vi "Init_Joint.vi"(7 "error in":errorcluster, 10 "X-CAN Session in":refnum<class "X-CAN.lvclass">) -> (0 "error out":errorcluster, 1 "Initial position":dbl[](array[numeric]), 2 "Init Position":T1(array[cluster]) {"Error Code" format="%b"; "ID" format="%x"}, 3 "X-CAN Session out":refnum<class "X-CAN.lvclass">)   [LabVIEW 2015]
uses:
  <vilib>/Stratom, Inc/X-CAN for myRIO (API)/X-CAN Class/X-CAN.lvclass
  <vilib>/Platform/TimedLoop/XDataNode/timing_clust.ctl
  <vilib>/Platform/TimedLoop/XDataNode/nitl_modes.ctl
  <vilib>/Platform/TimedLoop/XDataNode/wakeup.ctl
  <vilib>/Stratom, Inc/X-CAN for myRIO (API)/X-CAN Class/Type Definitions/CANFrame.ctl
  <vilib>/platform/TimedLoop/XDataNode/XDataNode.xnode
  <vilib>/Platform/TimedLoop/XDataNode/XDNodeRunTimeDep.lvlib
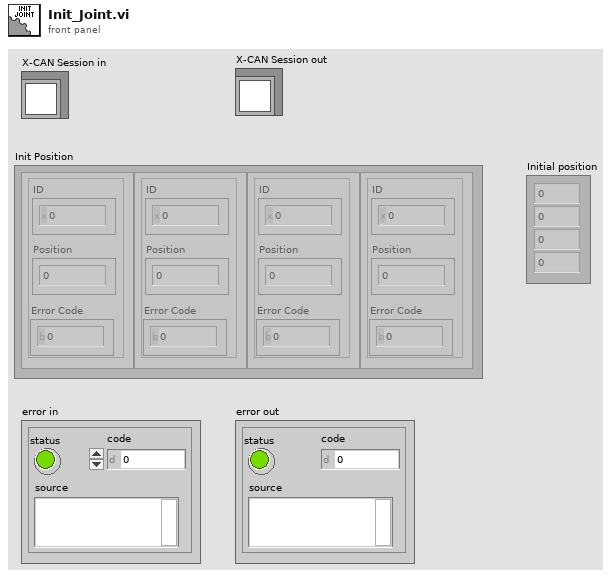
[diagram p1: front panel]
types:
  T1 = cluster{"ID":u8, "Position":u16, "Error Code":u8}[]
  T2 = typedef "XDNodeRunTimeDep.lvlib/timing_clust.ctl" = cluster{"Expected End [f-1]":u64, "Actual End [f-1]":u64, "Finished Late? [f-1]":bool, "Expected End [i-1]":u64, "Actual End [i-1]":u64, "Finished Late? [i-1]":bool, "Expected Start [i]":u64, "Actual Start [i]":u64, "Expected Start [f]":u64, "Actual Start [f]":u64, "Source Name":string, "Structure Name":string, "Period":i64, "Deadline":i64, "Offset":i64, "Start":i64, "Priority":i32, "Timeout":i32, "Mode":T3, "Wakeup Reason":T4, "Error":errorcluster, "Source Type":string, "Secondary Source Type":string, "Global End Time":u64, "Global Start Time":u64, "Frame Duration":u64, "Iteration Duration":u64, "Assigned CPU":i32, "I/O Scan Engine Mode":u32}
  T3 = typedef "XDNodeRunTimeDep.lvlib/nitl_modes.ctl" = enum32{"No Change", "Process missed periods, maintain original phase", "Discard missed periods, maintain original phase", "Process missed periods, ignore original phase", "Discard missed periods, ignore original phase"}
  T4 = typedef "XDNodeRunTimeDep.lvlib/wakeup.ctl" = enum32{"Normal", "Aborted", "Asynchronous wakeup", "Timing source error", "Timed loop error", "Timeout"}
  T5 = typedef "X-CAN.lvclass/CANFrame.ctl" = cluster{"identifier":u32, "extended?":bool, "echo?":bool, "payload":u8[], "timestamp":timestamp}
  T6 = cluster{"Error Code":u8, "Position":u16, "ID":u8}
  T7 = cluster{"ID":u8, "Position":u16, "Error Code":u8}
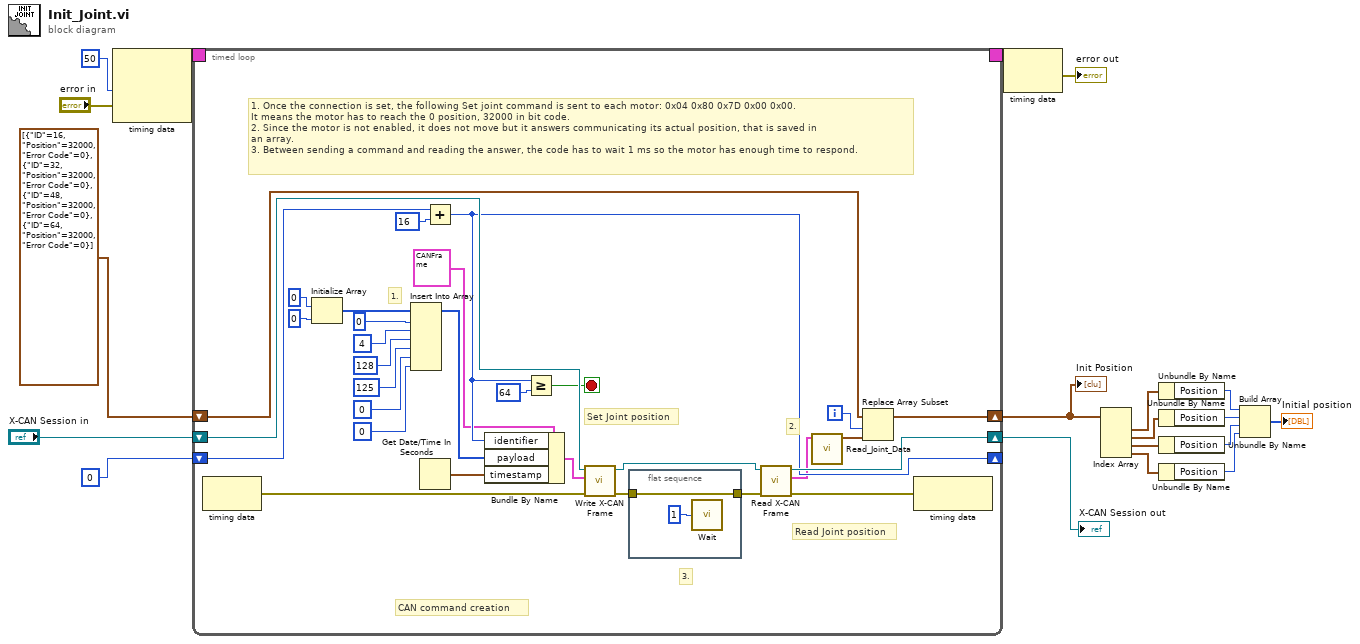
[diagram p0: block diagram]
diagram:
  n1 = node-c288(i64 50 ("Period"), "error in") -> (w19:T2)  [unwired: 1 in]
  n2 = timed-loop {
    timing: w19 -> [_]
    timing-out: [_] -> w18
    shift-right: [w49] -> w13
    shift-left: "X-CAN Session in" -> [w48]
    shift-right: [w47] -> _
    shift-left: u8 0 -> [w46]
    shift-right: [w45] -> w1
    shift-left: T1 [{"ID"=16, "Position"=32000, "Error Code"=0}, {"ID"=32, "Position"=32000, "Error Code"=0}, {"ID"=48, "Position"=32000, "Error Code"=0}, {"ID"=64, "Position"=32000, "Error Code"=0}] ("Array") -> [w44]
    i -> [w40]
    stop <- w41 stop-if-true
    # "1. Once the connection is set, the following Set joint command is sent to each motor: 0x04 0x80 0x7D 0x00 0x00.\nIt means the motor has to reach the 0 position, 32000 in bit code.\n2. Since the motor is not enabled, it does not move but it answers communicating its actual position, that is saved in\nan array.\n3. Between sending a command and reading the answer, the code has to wait 1 ms so the motor has enough time to respond."
    # "Read Joint position"
    # "3."
    # "2."
    # "1."
    # "Set Joint position"
    # "CAN command creation"
    n3 = node-c288() -> (w24:errorcluster)  [unwired: 1 in]
    n4 = Initialize Array(u16 0 ("element"), 0 ("dimension size")) -> (w34:u16[])
    n5 = Insert Into Array(array=w34, index=0, new element #1=u8 4 ("new element/subarray"), new element #2=u8 128 ("new element/subarray"), new element #3=u8 125 ("new element/subarray"), new element #4=u8 0 ("new element/subarray"), new element #5=u8 0 ("new element/subarray")) -> (w26:u16[])
    n6 = Get Date/Time In Seconds() -> (seconds since 1Jan1904=w38:timestamp)
    n7 = Add(x=w46, y=u8 16) -> (x+y=w47:u8)
    n8 = Bundle By Name(cluster=T5 {"identifier"=0, "extended?"=FALSE, "echo?"=FALSE, "payload"=[], "timestamp"=timestamp(0 s since 1904-01-01)} ("CAN Frame"), "identifier"=w47, "payload"=w26, "timestamp"=w38) -> (w31:T5)
    n9 = Greater Or Equal?(x=w47, y=u8 64) -> (x >= y?=w41:bool)
    n10 = call <vilib>:"Write X-CAN Frame.vi"("error in"=w24, "CAN Frame"=w31, "X-CAN Session in"=w48) -> ("error out"=w23:errorcluster, "X-CAN Session out"=w43:refnum<class "X-CAN.lvclass">)  [unwired: 7 in]
    n11 = flat-sequence {
      tunnel: w23 -> [w50]
      tunnel: [w50] -> w22
      frame #0 {
        n12 = call "Wait"("Count(mSec)"=u32 1) -> ()  [unwired: 1 out]
      }
    }
    n13 = call <vilib>:"Read X-CAN Frame.vi"("error in"=w22, "X-CAN Session in"=w43) -> ("error out"=w39:errorcluster, "CAN Frame"=w21:T5, "X-CAN Session out"=w49:refnum<class "X-CAN.lvclass">)  [unwired: 7 in]
    n14 = call "Read_Joint_Data.vi"("CAN Frame"=w21) -> ("Joint Position out"=w20:T6)  [unwired: 9 in, 1 out]
    n15 = Replace Array Subset(array=w44, new element=w20, index=w40) -> (w45:T1)
    n16 = node-c288(w39) -> ()  [unwired: 1 out]
  }
  "X-CAN Session out" <- w13
  "Init Position" <- w1
  n17 = node-c288(w18) -> (→"error out":errorcluster)
  n18 = Index Array(array=w1) -> (element #1=w10:T7, element #2=w9:T7, element #3=w8:T7, element #4=w7:T7)  [unwired: 4 in]
  n19 = Unbundle By Name(w10) -> ("Position"=w6:u16)
  n20 = Unbundle By Name(w9) -> ("Position"=w5:u16)
  n21 = Unbundle By Name(w8) -> ("Position"=w4:u16)
  n22 = Unbundle By Name(w7) -> ("Position"=w3:u16)
  n23 = Build Array(w6, w5, w4, w3) -> (→"Initial position":u16[])
